vi "Execution_Message_Act.vi"(7 "EVE reference in":refnum<data-value>, 8 "error in":errorcluster, 11 "ProcessStartedMessage in":refnum<class "ProcessStartedMessage.lvclass">) -> (0 "error out":errorcluster, 3 "ProcessStartedMessage out":refnum<class "ProcessStartedMessage.lvclass">)   [LabVIEW 2013, in "ProcessStartedMessage.lvclass"]
uses:
  ProcessStartedMessage.lvclass
  EVE/EVE.lvclass
  030 - EVENTS/05 - FromProcesses/FromProcessEvent.ctl
  030 - EVENTS/05 - FromProcesses/FromProcessesEventType.ctl
  030 - EVENTS/03 - ToMessageHandlerProcess/ToMessageHandlerEvent.ctl
  030 - EVENTS/03 - ToMessageHandlerProcess/enumMessageCriticity.ctl
  Messages.lvclass
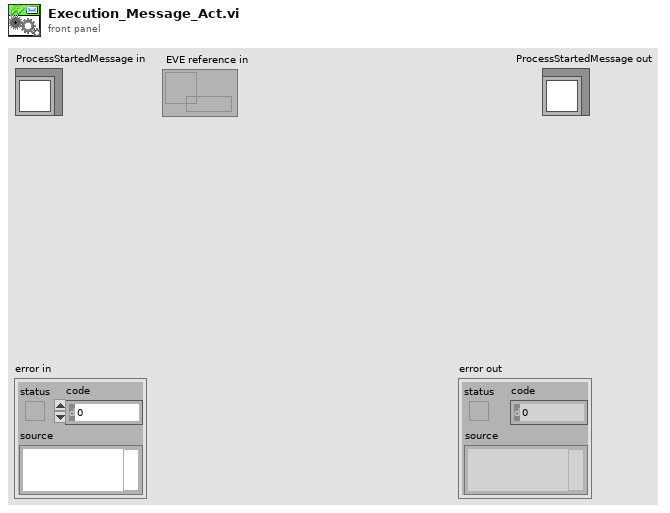
[diagram p1: front panel]
types:
  T1 = typedef "FromProcessesEventType.ctl" = enum16{"Started", "Autotest", "Ended"}
  T2 = typedef "FromProcessEvent.ctl" = cluster{"Command":T1, "Process path":path, "Message":T3, "Process Refnum":refnum<vi>}
  T3 = typedef "ToMessageHandlerEvent.ctl" = cluster{"date / time":timestamp, "Criticity":T4, "Emitter":string, "Message":string}
  T4 = typedef "enumMessageCriticity.ctl" = enum16{"No error", "Info", "Warning", "Error", "Fatal error"}
  T5 = typedef "usereventprio.ctl" = enum32{"high priority", "normal priority"}
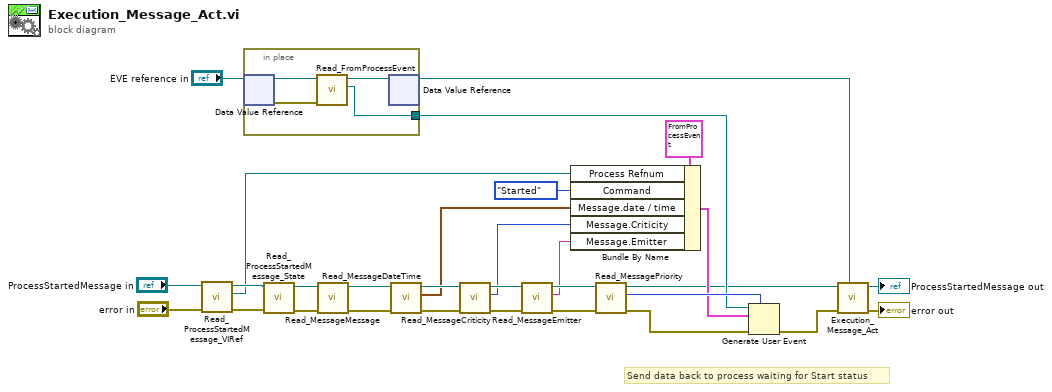
[diagram p0: block diagram]
diagram:
  # "Send data back to process waiting for Start status"
  n1 = call-dynamic "Read_ProcessStartedMessage_VIRef.vi"("error in (no error)"="error in", "ProcessStartedMessage in"="ProcessStartedMessage in") -> ("error out"=w19:errorcluster, "VI Refnum"=w25:refnum<vi>, "ProcessStartedMessage out"=w30:refnum<class "ProcessStartedMessage.lvclass">)  [unwired: 7 in]
  n2 = in-place {
    in-place-border: [w31] -> w21
    n3 = in-place-dvr #1("EVE reference in") -> (w34:refnum<class "EVE.lvclass">, w32:errorcluster)
    n4 = call "Read_FromProcessEvent.vi"("error in (no error)"=w32, "EVE.lvclass in"=w34) -> ("From Process Event"=w31:refnum<user-event>, "EVE.lvclass out"=w33:refnum<class "EVE.lvclass">)  [unwired: 7 in, 1 out]
    n5 = in-place-dvr #1(w33) -> (w6:refnum<data-value>)  [unwired: 1 out]
  }
  n6 = call-dynamic "Read_ProcessStartedMessage_State.vi"("error in (no error)"=w19, "ProcessStartedMessage in"=w30) -> ("error out"=w9:errorcluster, "ProcessStartedMessage out"=w11:refnum<class "ProcessStartedMessage.lvclass">)  [unwired: 7 in, 1 out]
  n7 = call-dynamic "Read_MessageMessage.vi"("error in (no error)"=w9, "Messages in"=w11) -> ("error out"=w8:errorcluster, "Messages out"=w10:refnum<class "ProcessStartedMessage.lvclass">)  [unwired: 7 in, 1 out]
  n8 = call-dynamic "Read_MessageDateTime.vi"("error in (no error)"=w8, "Messages in"=w10) -> ("error out"=w17:errorcluster, "date / time"=w18:timestamp, "Messages out"=w29:refnum<class "ProcessStartedMessage.lvclass">)  [unwired: 7 in]
  n9 = call-dynamic "Read_MessageCriticity.vi"("error in (no error)"=w17, "Messages in"=w29) -> ("error out"=w3:errorcluster, "Criticity"=w13:T4, "Messages out"=w15:refnum<class "ProcessStartedMessage.lvclass">)  [unwired: 7 in]
  n10 = call-dynamic "Read_MessageEmitter.vi"("error in (no error)"=w3, "Messages in"=w15) -> ("error out"=w16:errorcluster, "Emitter"=w12:string, "Messages out"=w14:refnum<class "ProcessStartedMessage.lvclass">)  [unwired: 7 in]
  n11 = Bundle By Name(cluster=T2 {"Command"=enum."Started", "Process path"=path "", "Message"={"date / time"=timestamp(0 s since 1904-01-01), "Criticity"=enum."No error", "Emitter"="", "Message"=""}, "Process Refnum"=refnum} ("event data"), "Process Refnum"=w25, "Command"=FromProcessesEventType."Started", "Message.date / time"=w18, "Message.Criticity"=w13, "Message.Emitter"=w12) -> (w24:T2)
  n12 = call-dynamic "Read_MessagePriority.vi"("error in (no error)"=w16, "Messages in"=w14) -> ("error out"=w1:errorcluster, "user event priority"=w28:T5, "Messages out"=w7:refnum<class "ProcessStartedMessage.lvclass">)  [unwired: 7 in]
  n13 = Generate User Event(priority (normal)=w28, user event=w21, event data cluster=w24, error in=w1) -> (error out=w2:errorcluster)  [unwired: 1 out]
  n14 = call-parent "Execution_Message_Act.vi"("EVE reference in"=w6, "error in (no error)"=w2, "Messages in"=w7) -> ("error out"=→"error out":errorcluster, "Messages out"=→"ProcessStartedMessage out":refnum<class "ProcessStartedMessage.lvclass">)  [unwired: 7 in]
